vi "Pemula 6.vi"() -> ()   [LabVIEW 2017]
uses:
  <vilib>/Instr/_visa.llb/VISA Configure Serial Port (Instr).vi
panel:
  out "concatenated string":string
  in  "stop":bool
  in  "VISA resource name":refnum<visa-resource-name>
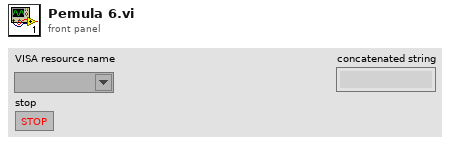
[diagram p1: front panel]
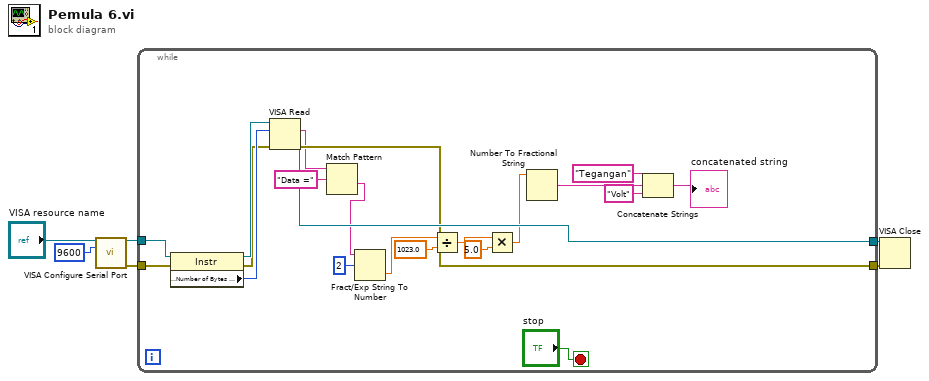
[diagram p0: block diagram]
diagram:
  n1 = call-poly "VISA Configure Serial Port"("VISA resource name"="VISA resource name", "baud rate (9600)"=9600) -> ("VISA resource name out"=w2:refnum<visa-resource-name>, "error out"=w4:errorcluster)  [unwired: 12 in]
  n2 = while {
    tunnel: [w24] -> w6
    tunnel: [w23] -> w5
    tunnel: w2 -> [w21]
    tunnel: w4 -> [w20]
    stop <- "stop" stop-if-true
    n3 = property class="Instr"(reference=w21, error in=w20) -> (reference out=w27:refnum<visa-resource-name>, error out=w25:errorcluster, "Serial Settings:Number of Bytes at Serial Port"=w26:u32)
    n4 = VISA Read(VISA resource name=w27, byte count=w26, error in (no error)=w25) -> (VISA resource name out=w24:refnum<visa-resource-name>, read buffer=w22:string, error out=w23:errorcluster)  [unwired: 1 out]
    n5 = Match Pattern(string=w22, regular expression="Data =") -> (after substring=w9:string)  [unwired: 1 in, 3 out]
    n6 = Fract/Exp String To Number(string=w9, offset=2) -> (number=w19:dbl)  [unwired: 2 in, 1 out]
    n7 = Divide(x=w19, y=1023.0) -> (x/y=w17:dbl)
    n8 = Multiply(x=w17, y=5.0) -> (x*y=w15:dbl)
    n9 = Number To Fractional String(number=w15) -> (F-format string=w13:string)  [unwired: 3 in]
    n10 = Concatenate Strings("Tegangan" ("string"), w13, "Volt" ("string")) -> (→"concatenated string":string)
  }
  n11 = VISA Close(VISA resource name=w6, error in (no error)=w5) -> ()  [unwired: 1 out]
